vi "MeasurementSpin2String_v02.vi"(0 "Program Spin Coater":T1(array[cluster]), 5 "Seconds to Spin Start":dbl[unit]=1.0, 7 "Seconds after Spin Stop":dbl[unit]=1.0, 9 "Spin Time":dbl[unit]=1.0, 11 "Time Detect":dbl[unit], 12 "Wavelength Detect":dbl[unit], 13 "Threshold":dbl) -> (4 "concatenated string":string)   [LabVIEW 2020]
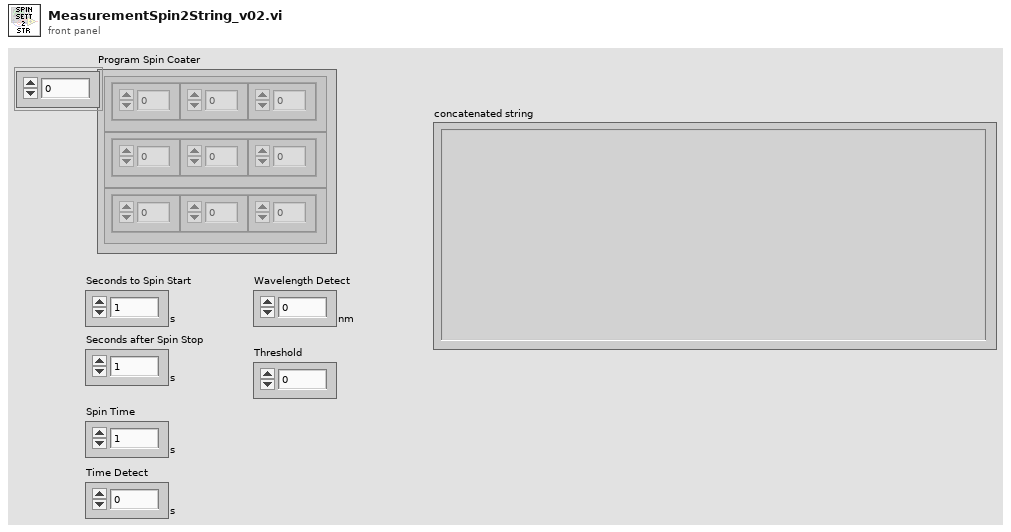
[diagram p1: front panel]
types:
  T1 = cluster{"Speed (rpm)":dbl, "Time (s)":dbl, "Acc (rpm/s)":dbl}[]
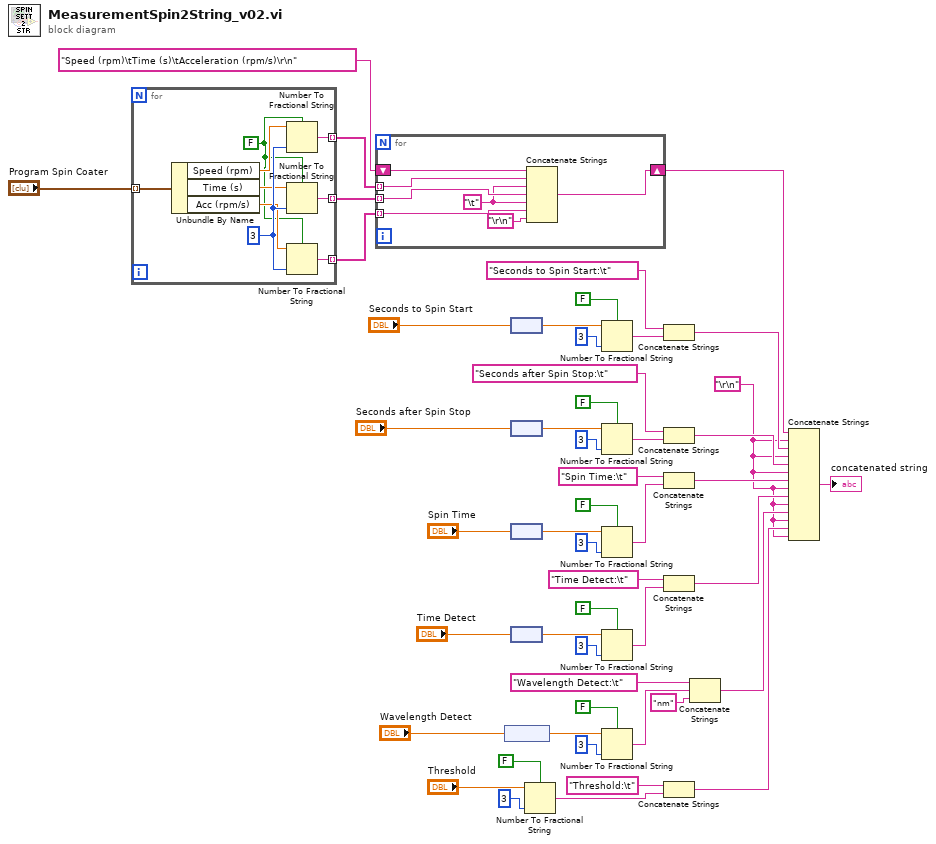
[diagram p0: block diagram]
diagram:
  w1 = "\r\n"
  n1 = for {
    tunnel: [w59] -> w49 mode=indexing
    tunnel: [w58] -> w47 mode=indexing
    tunnel: "Program Spin Coater" -> [w56] mode=indexing
    tunnel: [w53] -> w48 mode=indexing
    w57 = i16 3 ("precision (6)")
    w51 = FALSE ("use system decimal point (T)")
    n2 = Unbundle By Name(w56) -> ("Speed (rpm)"=w55:dbl, "Time (s)"=w54:dbl, "Acc (rpm/s)"=w52:dbl)
    n3 = Number To Fractional String(use system decimal point (T)=w51, number=w55, precision (6)=w57) -> (F-format string=w59:string)  [unwired: 1 in]
    n4 = Number To Fractional String(use system decimal point (T)=w51, number=w54, precision (6)=w57) -> (F-format string=w53:string)  [unwired: 1 in]
    n5 = Number To Fractional String(use system decimal point (T)=w51, number=w52, precision (6)=w57) -> (F-format string=w58:string)  [unwired: 1 in]
  }
  n6 = for {
    tunnel: w49 -> [w66] mode=indexing
    tunnel: w48 -> [w65] mode=indexing
    tunnel: w47 -> [w63] mode=indexing
    shift-right: [w61] -> w37
    shift-left: "Speed (rpm)\tTime (s)\tAcceleration (rpm/s)\r\n" -> [w62]
    w64 = "\t"
    n7 = Concatenate Strings(w62, w66, w64, w65, w64, w63, "\r\n") -> (w61:string)
  }
  n8 = node("Wavelength Detect") -> (w13:dbl)
  n9 = node("Seconds to Spin Start") -> (w42:dbl)
  n10 = node("Seconds after Spin Stop") -> (w44:dbl)
  n11 = node("Spin Time") -> (w35:dbl)
  n12 = node("Time Detect") -> (w30:dbl)
  n13 = Number To Fractional String(use system decimal point (T)=FALSE, number="Threshold", precision (6)=i16 3) -> (F-format string=w3:string)  [unwired: 1 in]
  n14 = Number To Fractional String(use system decimal point (T)=FALSE, number=w42, precision (6)=i16 3) -> (F-format string=w26:string)  [unwired: 1 in]
  n15 = Number To Fractional String(use system decimal point (T)=FALSE, number=w44, precision (6)=i16 3) -> (F-format string=w23:string)  [unwired: 1 in]
  n16 = Number To Fractional String(use system decimal point (T)=FALSE, number=w35, precision (6)=i16 3) -> (F-format string=w20:string)  [unwired: 1 in]
  n17 = Number To Fractional String(use system decimal point (T)=FALSE, number=w30, precision (6)=i16 3) -> (F-format string=w17:string)  [unwired: 1 in]
  n18 = Number To Fractional String(use system decimal point (T)=FALSE, number=w13, precision (6)=i16 3) -> (F-format string=w10:string)  [unwired: 1 in]
  n19 = Concatenate Strings("Seconds to Spin Start:\t", w26) -> (w25:string)
  n20 = Concatenate Strings("Seconds after Spin Stop:\t", w23) -> (w22:string)
  n21 = Concatenate Strings("Spin Time:\t", w20) -> (w19:string)
  n22 = Concatenate Strings("Time Detect:\t", w17) -> (w16:string)
  n23 = Concatenate Strings("Threshold:\t", w3) -> (w2:string)
  n24 = Concatenate Strings("Wavelength Detect:\t", w10, "nm" ("string")) -> (w8:string)
  n25 = Concatenate Strings(w37, w1, w25, w1, w22, w1, w19, w1, w16, w1, w8, w1, w2, w1) -> (→"concatenated string":string)
